vi "Write Event Fired Msg.vi"(10 "Event Source.lvlib:Event Fired Msg.lvclass":refnum<class "Event Fired Msg.lvclass">=refnum, 11 "Event Source in":refnum<class "Event Source.lvclass">) -> (3 "Event Source out":refnum<class "Event Source.lvclass">)   [LabVIEW 2016, in "Event Source.lvlib" / "Event Source.lvclass"]
uses:
  <vilib>/NI/Event Source Actor/Event Source/Event Source/Event Source.lvclass
  Google Drive/MyCode/.Event Source/Event Source/Event Source Messages/Event Fired Msg/Event Fired Msg.lvclass
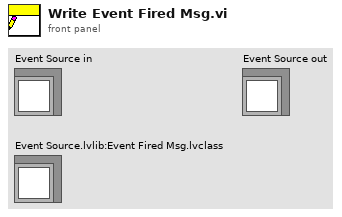
[diagram p1: front panel]
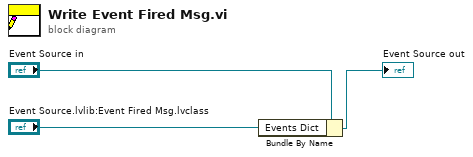
[diagram p0: block diagram]
diagram:
  n1 = Bundle By Name(cluster="Event Source in", "Events Dict"="Event Source.lvlib:Event Fired Msg.lvclass") -> (→"Event Source out":refnum<class "Event Source.lvclass">)
